vi "Format Date-Time for Table.vi"(11 "Time Stamp":timestamp) -> (3 "String":string)   [LabVIEW 2011]
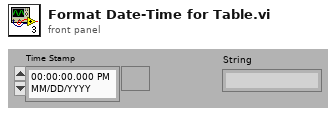
[diagram p1: front panel]
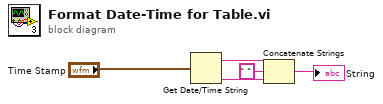
[diagram p0: block diagram]
diagram:
  n1 = Get Date/Time String(seconds (now)="Time Stamp") -> (date string=w4:string, time string=w3:string)  [unwired: 2 out]
  n2 = Concatenate Strings(w4, " " ("string"), w3) -> (→"String":string)
